vi "Entrada String con salida Double.vi"(1 "stop":bool, 2 "Palabra":string) -> (0 "Numero":dbl)   [LabVIEW 2021]
doc: "En este programa, escribes una cadena de caracterés tipo string, correspondiendo a un numero entre 0 y 9, entregando como resultaddo el nummero con el que se escribió, es importante no equivocarse con la escritura del numero en cuestión. Es indiferente por cualquier mayúscula o minúscula presente\n\nElaboró: Mendoza Meza Manuel Everardo"
panel:
  # "Mendoza Meza Manuel Everardo"
  # "Entrada String con salida Numerica"
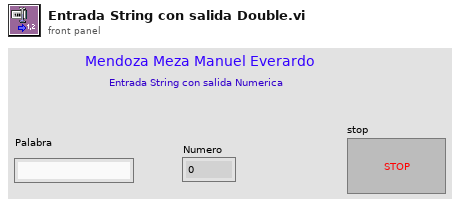
[diagram p1: front panel]
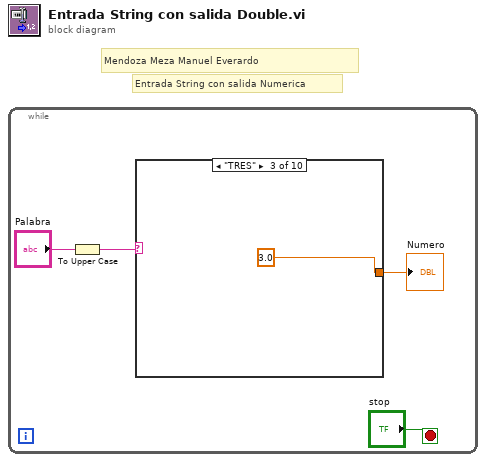
[diagram p0: block diagram]
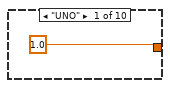
[diagram p2: hidden frame]
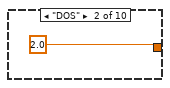
[diagram p3: hidden frame]
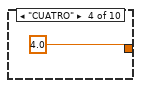
[diagram p4: hidden frame]
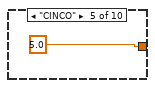
[diagram p5: hidden frame]
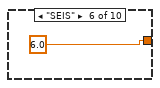
[diagram p6: hidden frame]
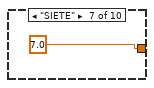
[diagram p7: hidden frame]
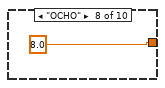
[diagram p8: hidden frame]
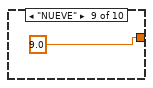
[diagram p9: hidden frame]
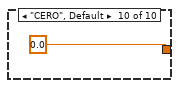
[diagram p10: hidden frame]
diagram:
  # "Entrada String con salida Numerica"
  # "Mendoza Meza Manuel Everardo"
  n1 = while {
    stop <- "stop" stop-if-true
    n2 = To Upper Case(1:"Palabra") -> (0:w2:string)
    n3 = case shown="\"TRES\"" w2 {
      tunnel: [1.0 2.0 3.0 4.0 5.0 6.0 7.0 8.0 9.0 0.0] -> w1
      frame "UNO" {
      }
      frame "DOS" {
      }
      frame "TRES" {
      }
      frame "CUATRO" {
      }
      frame "CINCO" {
      }
      frame "SEIS" {
      }
      frame "SIETE" {
      }
      frame "OCHO" {
      }
      frame "NUEVE" {
      }
      frame "CERO", Default {
      }
    }
    "Numero" <- w1
  }
